vi "oa_Shift and Low Pass Filter (N Channels, Obsolete).vi"(0 "input signal":dbl[][](array[numeric]) format="%.2f", 1 "reset? (F)":bool, 5 "t0":dbl, 7 "center":dbl, 9 "decimation factor":u32, 11 "error in (no error)":errorcluster, 12 "new dt":dbl) -> (4 "envelope signal":dbl[][](array[numeric]) format="%.2f", 6 "t0 out":dbl, 15 "error out":errorcluster)   [LabVIEW 2017]
uses:
  <vilib>/addons/Sound and Vibration/Order Analysis/Adv Resampling/OAT Single Stage Decimation with IC.vi
  <vilib>/addons/Sound and Vibration/Order Analysis/Resample Order Tracking/SubVIs/OAT CIC Decimation.vi
  <vilib>/addons/Sound and Vibration/Order Analysis/Resample Order Tracking/SubVIs/oa_Interpolate Zeros Between Samples.vi
  <vilib>/addons/Sound and Vibration/Order Analysis/Resample Order Tracking/SoundVib_Resampling.lvlib
  <vilib>/Analysis/NI_AALPro.lvlib
  <vilib>/addons/Sound and Vibration/Order Analysis/Fault Analysis/SoundVib_FaultAnalysis.lvlib
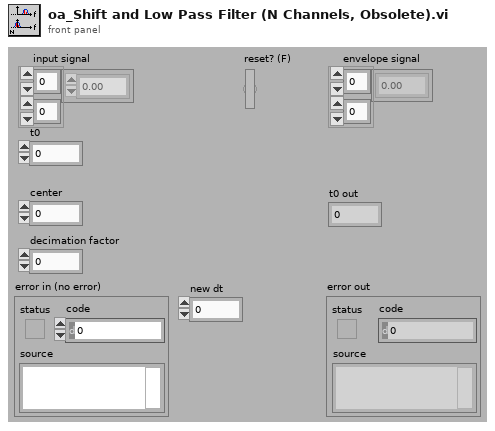
[diagram p1: front panel]
types:
  T1 = typedef "OAT Decimation Filter.ctl" = cluster{"coefficients":dbl[], "factor":i32}
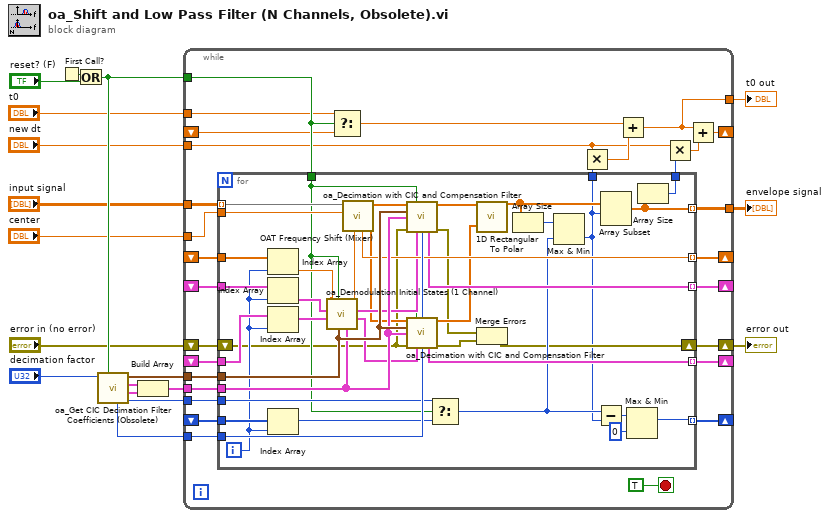
[diagram p0: block diagram]
diagram:
  n1 = First Call?() -> (First Call?: T/F=w18:bool)
  n2 = Or(x=w18, y="reset? (F)") -> (x .or. y?=w16:bool)
  n3 = call <vilib>:"oa_Get CIC Decimation Filter Coefficients (Obsolete).vi"("reset? (True)"=w16, "decimation/interpolation factor"="decimation factor") -> ("delay"=w10:i32, "lp filter settings"=w13:T1, "compensation filter settings"=w14:T1, "CIC Settings"=w15:cluster{"Numeric":i32, i32, i32}, "interpolation factor"=w11:i32)  [unwired: 5 in]
  n4 = Build Array(w14, w13) -> (w12:T1[])
  n5 = while {
    tunnel: w16 -> [w29]
    tunnel: w15 -> [w47]
    tunnel: w12 -> [w46]
    tunnel: w11 -> [w45]
    tunnel: w10 -> [w44]
    tunnel: "center" -> [w43]
    tunnel: "input signal" -> [w42]
    shift-right: [w40] -> _
    shift-left: _ -> [w36]
    shift-right: [w39] -> _
    shift-left: _ -> [w35]
    shift-right: [w38] -> _
    shift-left: _ -> [w34]
    shift-right: [w37] -> _
    shift-left: _ -> [w33]
    shift-right: [w31] -> w1
    shift-left: "error in (no error)" -> [w32]
    tunnel: [w30] -> w6
    shift-right: [w20] -> _
    shift-left: _ -> [w24]
    tunnel: "t0" -> [w28]
    tunnel: "new dt" -> [w23]
    tunnel: [w19] -> w3
    stop <- TRUE stop-if-true
    n6 = for {
      tunnel: w47 -> [w86]
      tunnel: w46 -> [w85]
      tunnel: w45 -> [w84]
      tunnel: w44 -> [w83]
      tunnel: w43 -> [w82]
      tunnel: w42 -> [w53] mode=indexing
      tunnel: [w81] -> w40 mode=indexing
      tunnel: [w80] -> w39 mode=indexing
      tunnel: [w79] -> w38 mode=indexing
      tunnel: [w78] -> w37 mode=indexing
      tunnel: w36 -> [w61]
      tunnel: w35 -> [w59]
      tunnel: w34 -> [w57]
      tunnel: w33 -> [w55]
      shift-right: [w63] -> w31
      shift-left: w32 -> [w48]
      tunnel: [w50] -> w30 mode=indexing
      tunnel: w29 -> [w52]
      tunnel: [w51] -> w26
      tunnel: [w49] -> w22
      i -> [w54]
      n7 = Index Array(array=w61, index=w54) -> (element=w62:dbl)
      n8 = Index Array(array=w59, index=w54) -> (element=w60:cluster{cluster{dbl[]}, cluster{dbl[]}[]})
      n9 = Index Array(array=w57, index=w54) -> (element=w58:cluster{cluster{dbl[]}, cluster{dbl[]}[]})
      n10 = Index Array(array=w55, index=w54) -> (element=w56:i32)
      n11 = call <vilib>:"oa_Demodulation Initial States (1 Channel).vi"("filters"=w85, "CIC filter settings"=w86, "reset? (F)"=w52, "imaginary state in"=w58, "real state in"=w60, "phase in"=w62) -> ("imaginary state out"=w73:cluster{cluster{dbl[]}, cluster{dbl[]}[]}, "real state out"=w74:cluster{cluster{dbl[]}, cluster{dbl[]}[]}, "phase out"=w77:dbl)  [unwired: 3 in]
      n12 = call <vilib>:"OAT Frequency Shift (Mixer).vi"("initial phase"=w77, "fc"=w82, "X"=w53) -> ("imaginary"=w70:dbl[], "real"=w67:dbl[], "final phase"=w81:dbl)  [unwired: 6 in]
      n13 = call <vilib>:"oa_Decimation with CIC and Compensation Filter.vi"("x[n]"=w67, "reset? (True)"=w52, "CIC decimation setting"=w86, "decimation filters"=w85, "error in (no error)"=w48, "statein"=w74, "interpolation factor"=w84) -> ("x[n] out"=w65:dbl[], "state out"=w80:cluster{cluster{dbl[]}, cluster{dbl[]}[]}, "error out"=w66:errorcluster)  [unwired: 6 in]
      n14 = call <vilib>:"oa_Decimation with CIC and Compensation Filter.vi"("x[n]"=w70, "reset? (True)"=w52, "CIC decimation setting"=w86, "decimation filters"=w85, "error in (no error)"=w48, "statein"=w73, "interpolation factor"=w84) -> ("x[n] out"=w71:dbl[], "state out"=w79:cluster{cluster{dbl[]}, cluster{dbl[]}[]}, "error out"=w69:errorcluster)  [unwired: 6 in]
      n15 = Select(t=w83, s=w52, f=w56) -> (s? t:f=w72:i32)
      n16 = call <vilib>:"1D Rectangular To Polar.vi"("X"=w65, "Y"=w71) -> ("Magnitude"=w64:dbl[])  [unwired: 2 out]
      n17 = Merge Errors(w66, w69) -> (w63:errorcluster)
      n18 = Array Size(array=w64) -> (size(s)=w68:i32)
      n19 = Max & Min(x=w68, y=w72) -> (min(x,y)=w51:i32)  [unwired: 1 out]
      n20 = Subtract(x=w72, y=w51) -> (x-y=w76:i32)
      n21 = Array Subset(array=w64, index=w51) -> (w50:dbl[])  [unwired: 1 in]
      n22 = Max & Min(x=w76, y=0) -> (max(x,y)=w78:i32)  [unwired: 1 out]
      n23 = Array Size(array=w50) -> (size(s)=w49:i32)
    }
    n24 = Select(t=w28, s=w29, f=w24) -> (s? t:f=w27:dbl)
    n25 = Multiply(x=w23, y=w26) -> (x*y=w25:dbl)
    n26 = Add(x=w27, y=w25) -> (x+y=w19:dbl)
    n27 = Multiply(x=w23, y=w22) -> (x*y=w21:dbl)
    n28 = Add(x=w19, y=w21) -> (x+y=w20:dbl)
  }
  "envelope signal" <- w6
  "t0 out" <- w3
  "error out" <- w1
